vi "Throw Error.vi"(8 "Error In":errorcluster, 10 "Show Call Chain? (Def=T)":bool=TRUE, 11 "Error Message":string) -> (0 "Error Out":errorcluster)   [LabVIEW 2023, in "Error Manager.lvlib"]
doc: "This VI throws a custom, user-generated error if and only if there is no error at the \"Error In\" input.\n\nIn other words, this VI never overwrites an existing error. This behaviour is desirable in most cases."
uses:
  Error Manager.lvlib
panel:
  # "Input\nInputs to the VI"
  # "Development\nControls or indicators that are useful for development or testing, but which are not outputs of the VI."
  # "Output\nOutputs of the VI"
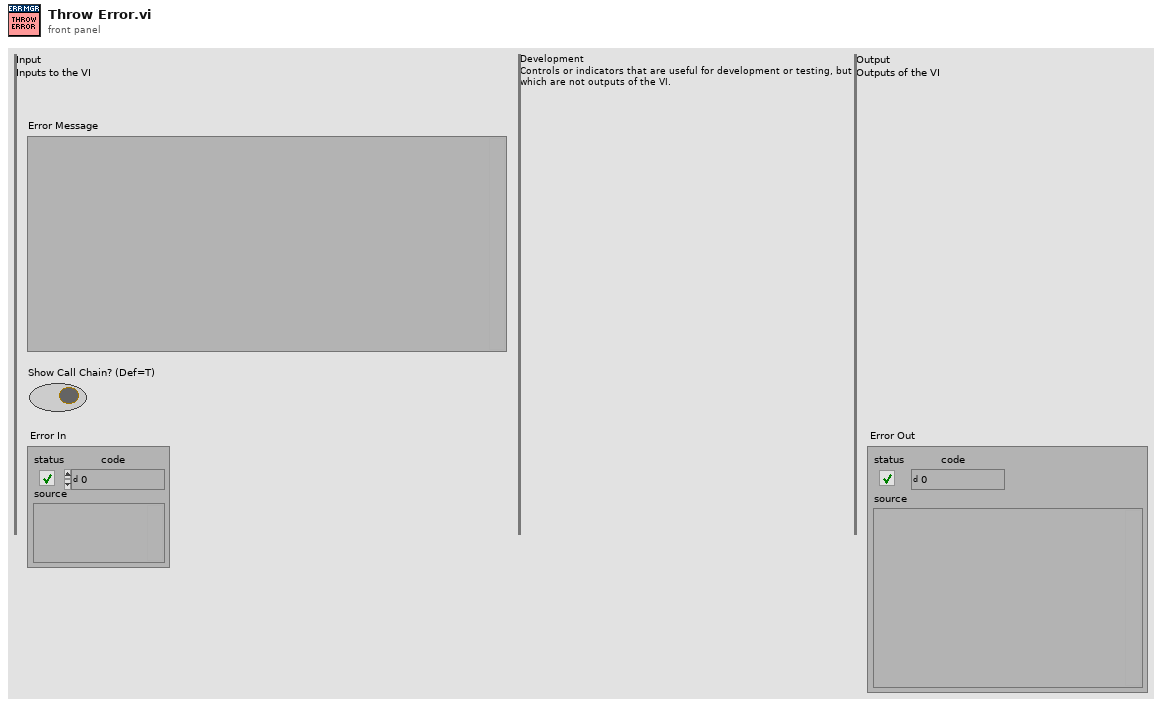
[diagram p1: front panel]
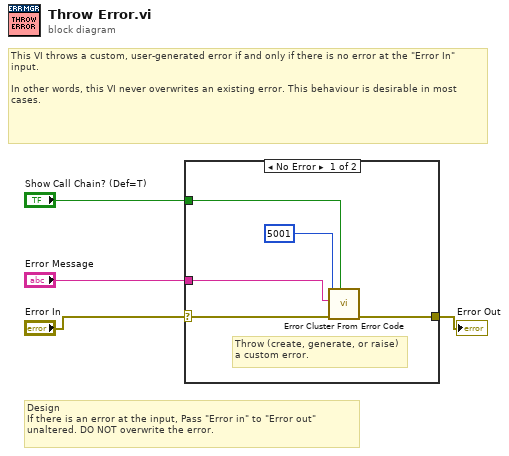
[diagram p0: block diagram]
diagram:
  # "This VI throws a custom, user-generated error if and only if there is no error at the \"Error In\" input.\n\nIn other words, this VI never overwrites an existing error. This behaviour is desirable in most cases."
  # "Design\nIf there is an error at the input, Pass \"Error in\" to \"Error out\" unaltered. DO NOT overwrite the error."
  n1 = case shown="No Error" "Error In" {
    selector: "Error In" -> [w6 w10]
    tunnel: [w9 w10] -> w4
    tunnel: "Show Call Chain? (Def=T)" -> [w8 _]
    tunnel: "Error Message" -> [w7 _]
    frame No Error {
      # "Throw (create, generate, or raise) a custom error."
      n2 = call <vilib>:"Error Cluster From Error Code.vi"("show call chain? (False)"=w8, "error in (no error)"=w6, "error message (\"\")"=w7, "error code (0)"=5001) -> ("error out"=w9:errorcluster)  [unwired: 5 in]
    }
    frame Error {
    }
  }
  "Error Out" <- w4
